vi "Read Connect Parameter.vi"(8 "error in (no error)":errorcluster, 11 "IOCard in":refnum<class "IOCard.lvclass">) -> (0 "error out":errorcluster, 2 "Connect Parameter":T2={"IO Card Type"=enum."None", "IOType"=enum."Output", "CardNumber"=0, "ConnectAct"=FALSE, "IP"=""}, 3 "IOCard out":refnum<class "IOCard.lvclass">)   [LabVIEW 2019, in "IOCard.lvclass"]
uses:
  IOCard.lvclass
  IO_VI/IOCtrl/Ctrl/IO Card_Type.ctl
  IOCard.lvclass/IOCard.ctl
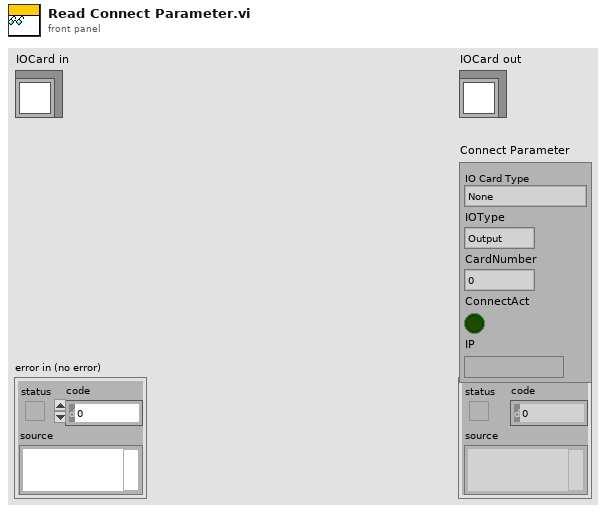
[diagram p1: front panel]
types:
  T1 = typedef "IO Card_Type.ctl" = enum16{"None", "Unidaq32", "6480", "2410C-64", "Zan", "DMC1000B", "16InOut", "Robot", "DMC3600"}
  T2 = cluster{"IO Card Type":T1, "IOType":enum16{"Input", "Output"}, "CardNumber":i32, "ConnectAct":bool, "IP":string}
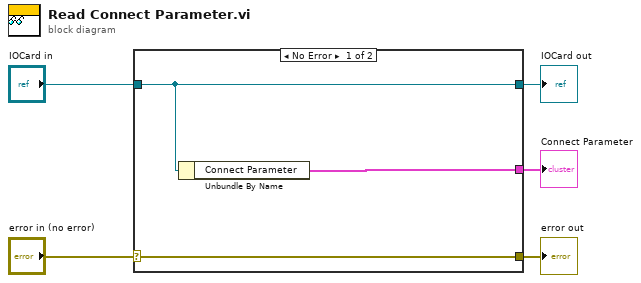
[diagram p0: block diagram]
diagram:
  n1 = case shown="No Error" "error in (no error)" {
    selector: "error in (no error)" -> [w8 w9]
    tunnel: [w8 w9] -> w4
    tunnel: [w7 w10] -> w2
    tunnel: "IOCard in" -> [w7 w10]
    tunnel: [w6 _] -> w1
    frame No Error {
      n2 = Unbundle By Name(w7) -> ("Connect Parameter"=w6:T2)
    }
    frame Error {
    }
  }
  "error out" <- w4
  "IOCard out" <- w2
  "Connect Parameter" <- w1
